vi "Factorial.vi"() -> ()   [LabVIEW 2022 SP3]
panel:
  out "Factorial":i32
  in  "Numeric":i32
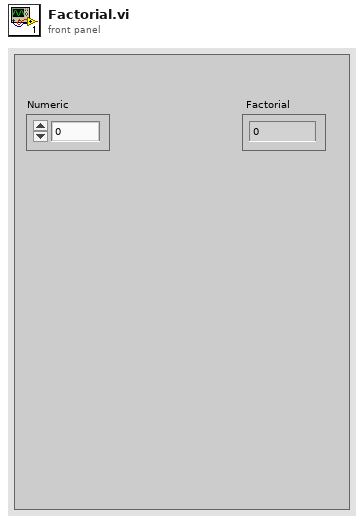
[diagram p1: front panel]
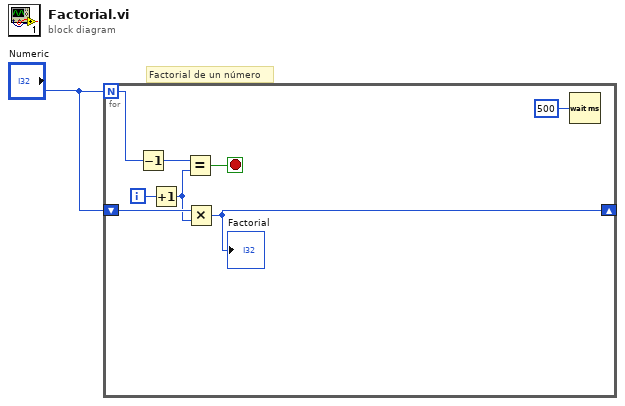
[diagram p0: block diagram]
diagram:
  # "Factorial de un número"
  n1 = for {
    N: "Numeric" -> [w5]
    shift-right: [w8] -> _
    shift-left: "Numeric" -> [w7]
    i -> [w9]
    stop <- w2 stop-if-true
    n2 = Decrement(x=w5) -> (x-1=w4:i32)
    n3 = Increment(x=w9) -> (x+1=w3:i32)
    n4 = Equal?(x=w4, y=w3) -> (x = y?=w2:bool)
    n5 = Multiply(x=w7, y=w3) -> (x*y=w8:i32)
    "Factorial" <- w8
    n6 = Wait (ms)(milliseconds to wait=u32 500) -> ()  [unwired: 1 out]
  }
